vi "database path.vi"(7 "数据库类型":T1, 9 "Password":string, 10 "ping":bool, 11 "database":string="database1") -> (2 "Connection information":string, 3 "Path out":string)   [LabVIEW 2016]
uses:
  Access/Access Lib.lvlib
  SQLite/SQLite Lib.lvlib
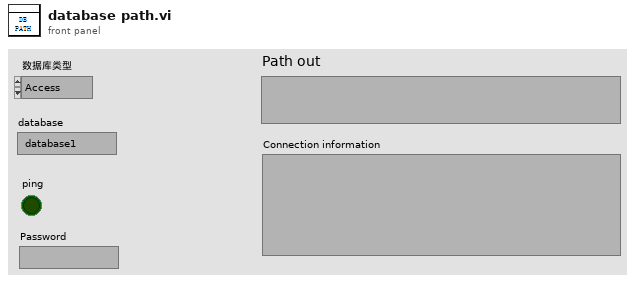
[diagram p1: front panel]
types:
  T1 = typedef "数据库类型.ctl" = enum16{"Access", "SQLite"}
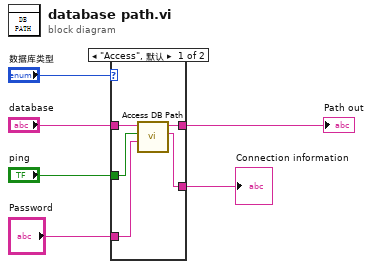
[diagram p0: block diagram]
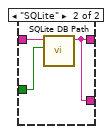
[diagram p2: hidden frame]
diagram:
  n1 = case shown="\"Access\", 默认" "数据库类型" {
    tunnel: [w11 w12] -> w3
    tunnel: "database" -> [w10 w14]
    tunnel: "ping" -> [w9 w13]
    tunnel: [w8 w12] -> w2
    tunnel: "Password" -> [w7 _]
    frame "Access", Default {
      n2 = call "Access DB Path.vi"("Password"=w7, "ping"=w9, "database"=w10) -> ("Connection information"=w8:string, "Path out"=w11:string)  [unwired: 7 in]
    }
    frame "SQLite" {
      n3 = call "SQLite DB Path.vi"("ping"=w13, "database"=w14) -> ("Path out"=w12:string)  [unwired: 9 in]
    }
  }
  "Path out" <- w3
  "Connection information" <- w2
